vi "Write supported targets.vi"(8 "error in":errorcluster, 10 "supported targets":T1[](array[typedef]), 11 "DecideProjectFeatures in":refnum<class "DCAFConfigurablePluginDecideFeatures.lvclass">) -> (0 "error out":errorcluster, 3 "DecideProjectFeatures out":refnum<class "DCAFConfigurablePluginDecideFeatures.lvclass">)   [LabVIEW 2013, in "DCAFConfigurablePluginDecideFeatures.lvclass"]
uses:
  DCAFConfigurablePluginDecideFeatures.lvclass
  <vilib>/NI/Tag Bus Module Framework/root configuration/Target Types.ctl
  DCAFConfigurablePluginDecideFeatures.lvclass/DCAFConfigurablePluginDecideFeatures.ctl
  <vilib>/NI/Tag Bus Module Framework/root configuration/TBM configuration.lvclass
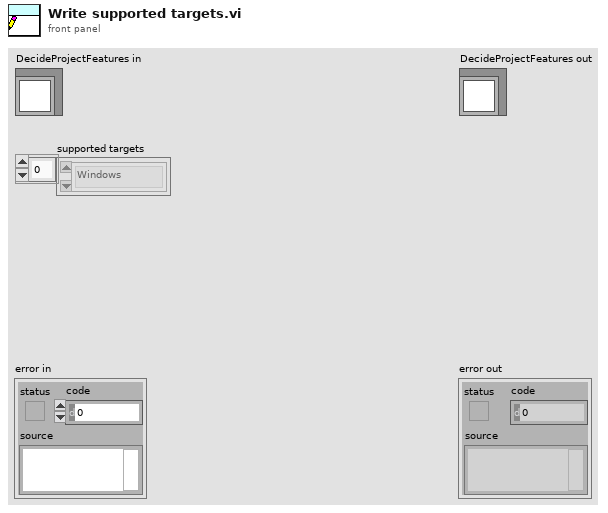
[diagram p1: front panel]
types:
  T1 = typedef "TBM configuration.lvclass/Target Types.ctl" = enum16{"Windows", "Mac", "Linux", "Linux RT ARM", "VxWorks", "Pharlap", "Other", "Linux RT x64"}
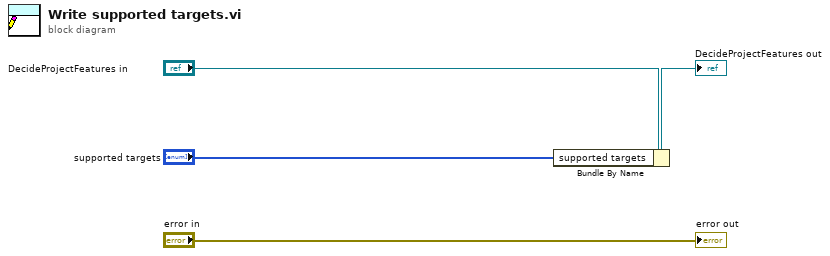
[diagram p0: block diagram]
diagram:
  n1 = Bundle By Name(cluster="DecideProjectFeatures in", "supported targets"="supported targets") -> (→"DecideProjectFeatures out":refnum<class "DCAFConfigurablePluginDecideFeatures.lvclass">)
  "error out" <- "error in"
